vi "LS370_setup.vi"   [LabVIEW 2016]
uses:
  Instrument_Setup.vi
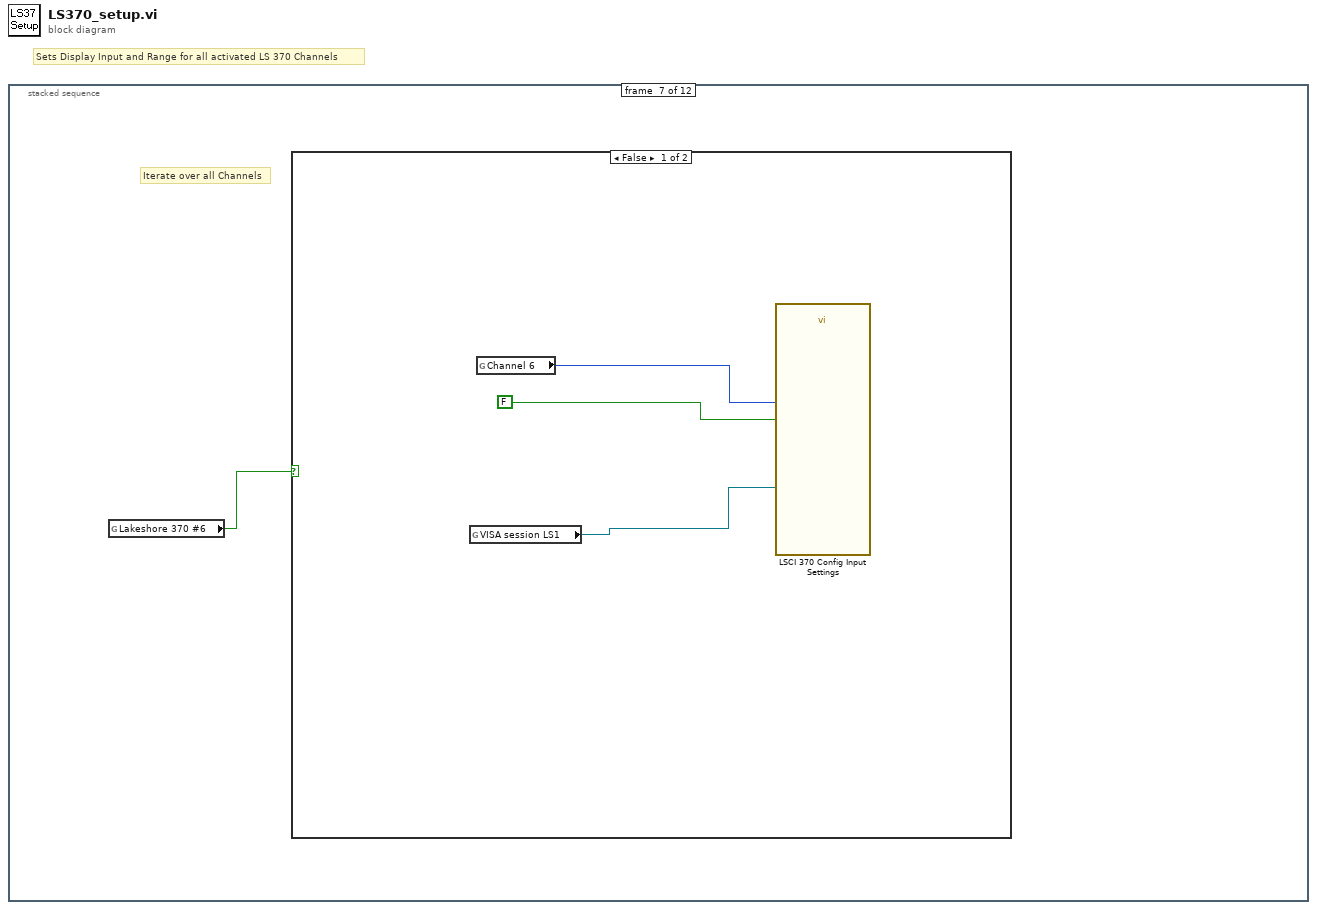
[diagram p0: block diagram]
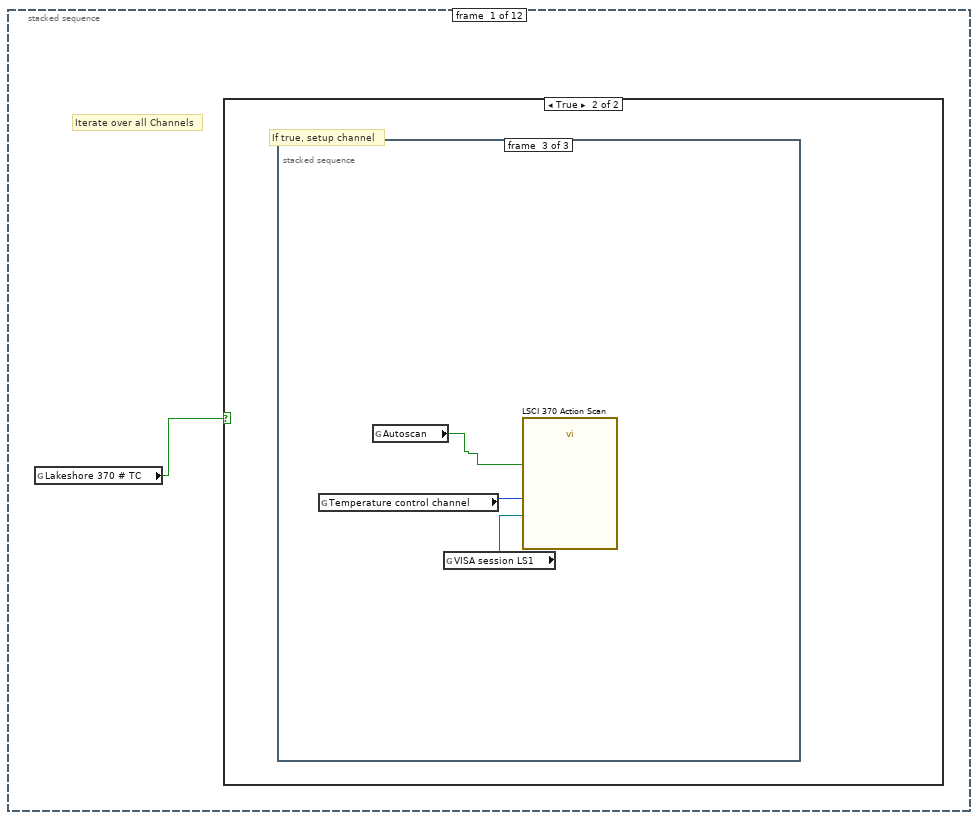
[diagram p2: hidden frame]
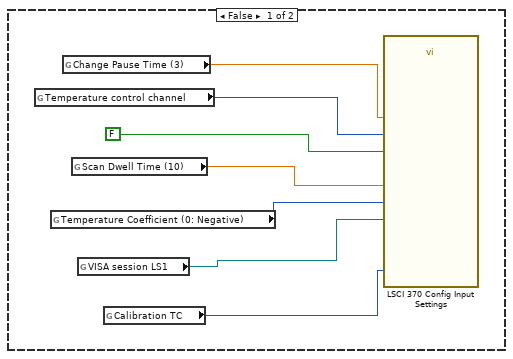
[diagram p3: hidden frame]
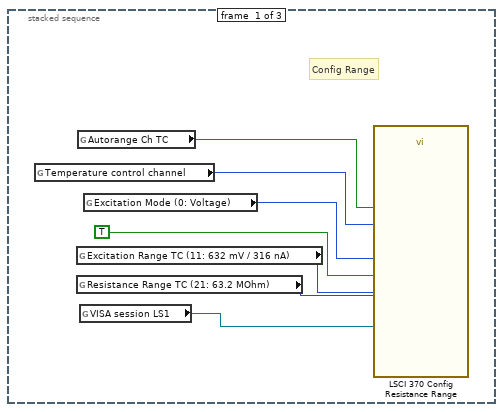
[diagram p4: hidden frame]
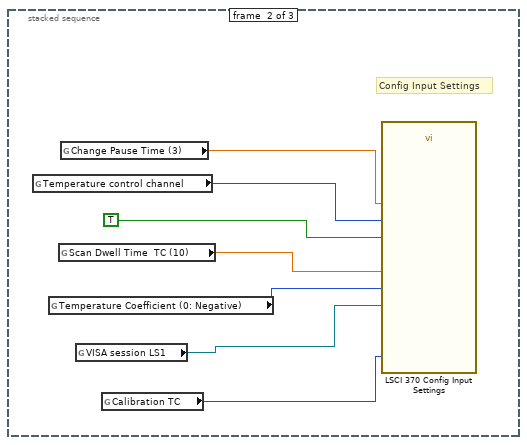
[diagram p5: hidden frame]
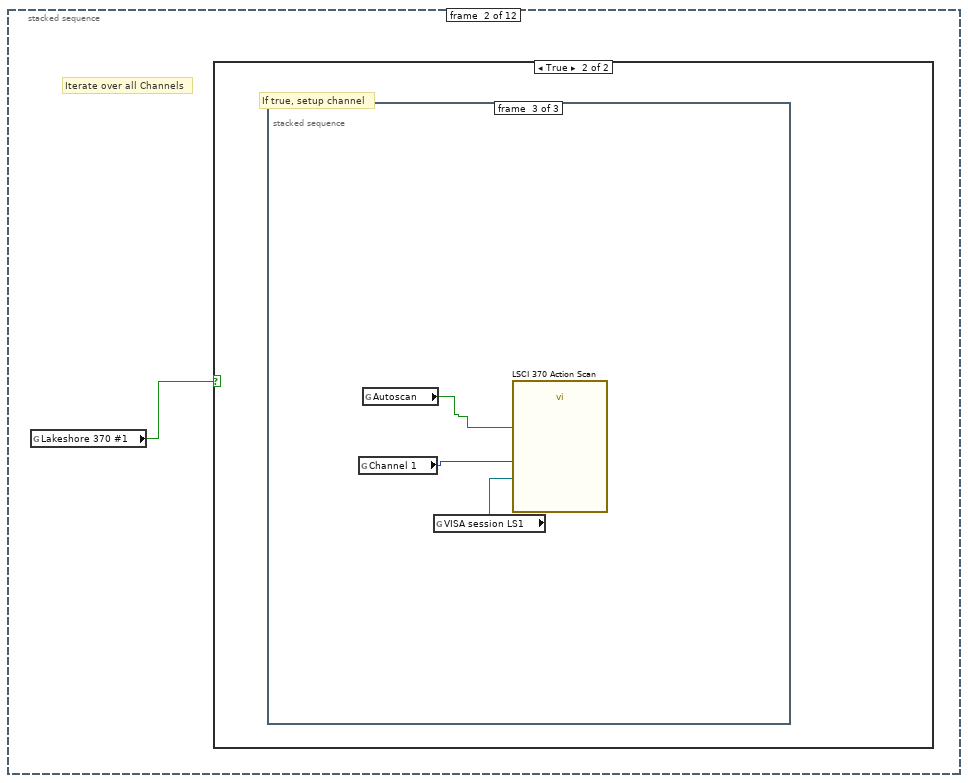
[diagram p6: hidden frame]
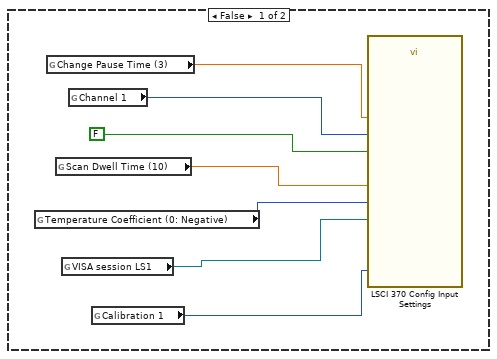
[diagram p7: hidden frame]
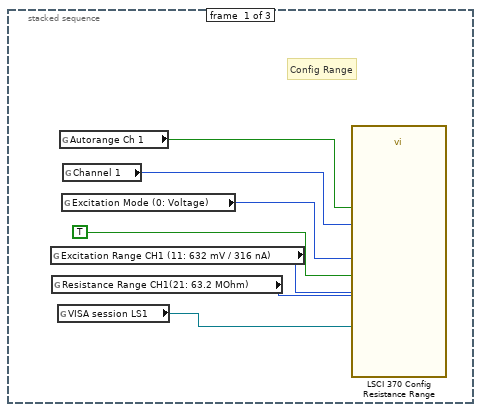
[diagram p8: hidden frame]
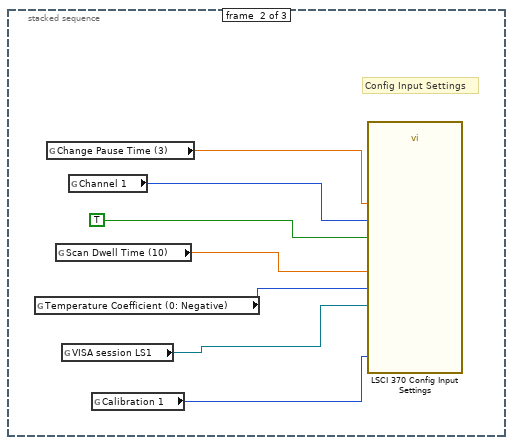
[diagram p9: hidden frame]
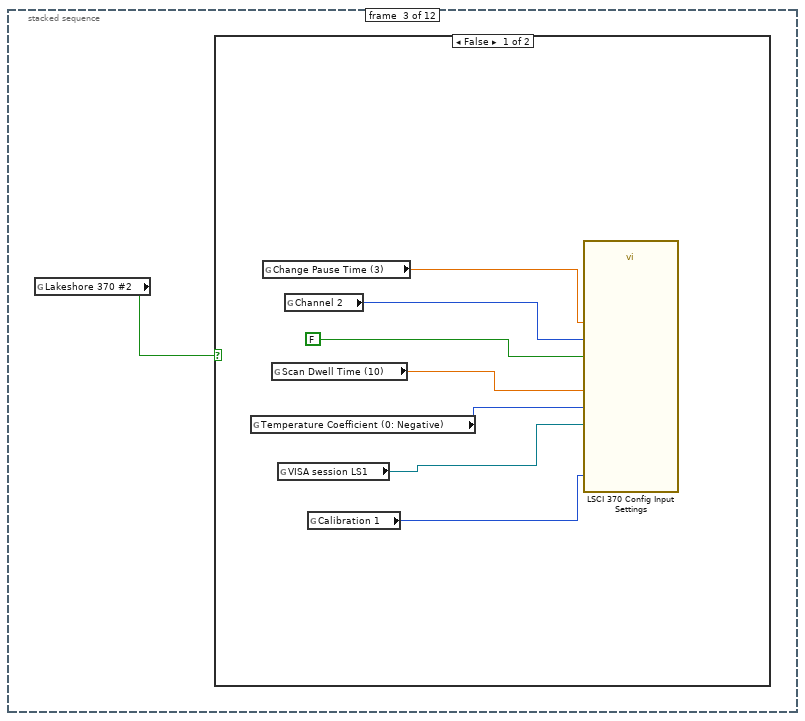
[diagram p10: hidden frame]
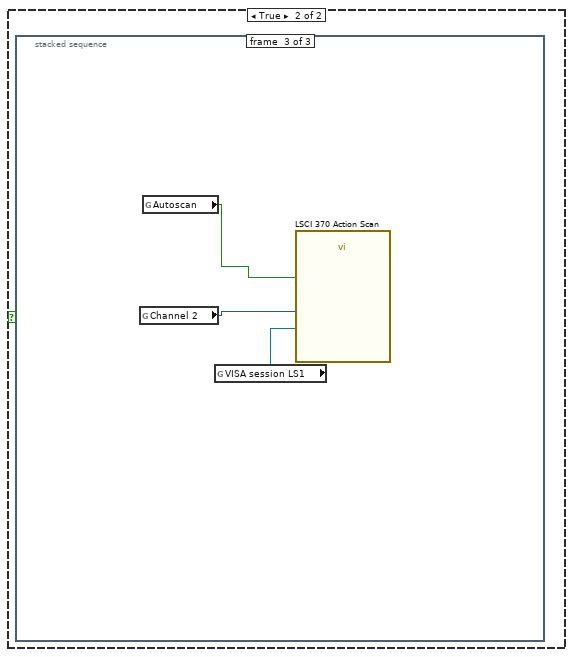
[diagram p11: hidden frame]
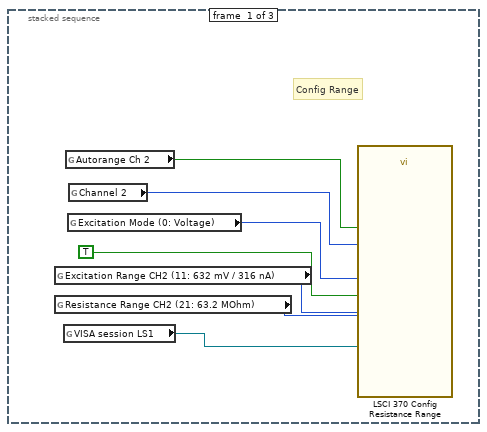
[diagram p12: hidden frame]
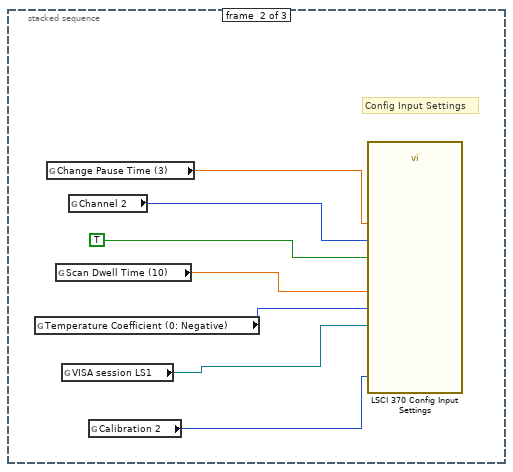
[diagram p13: hidden frame]
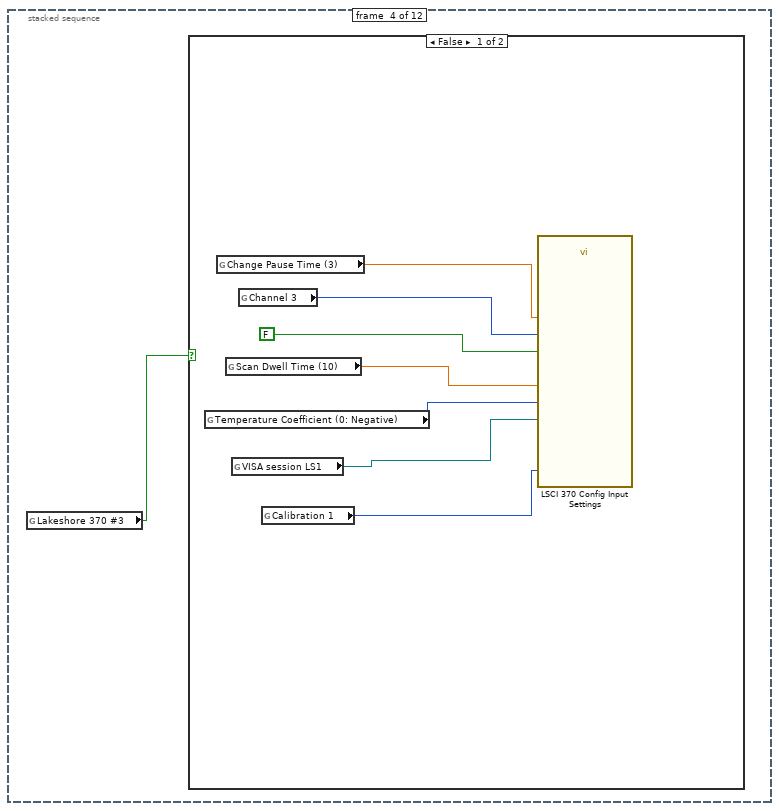
[diagram p14: hidden frame]
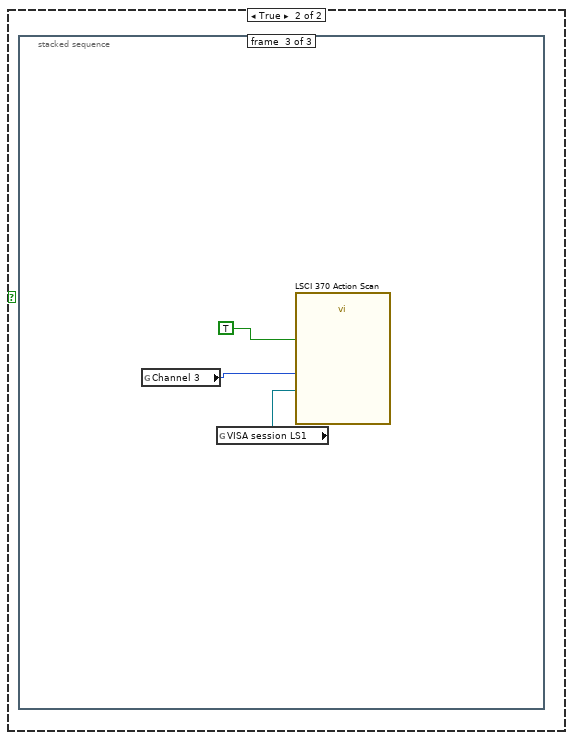
[diagram p15: hidden frame]
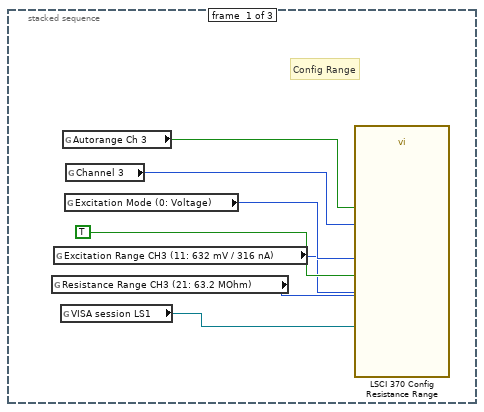
[diagram p16: hidden frame]
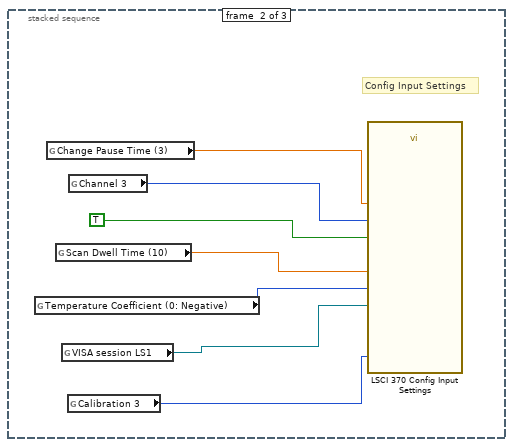
[diagram p17: hidden frame]
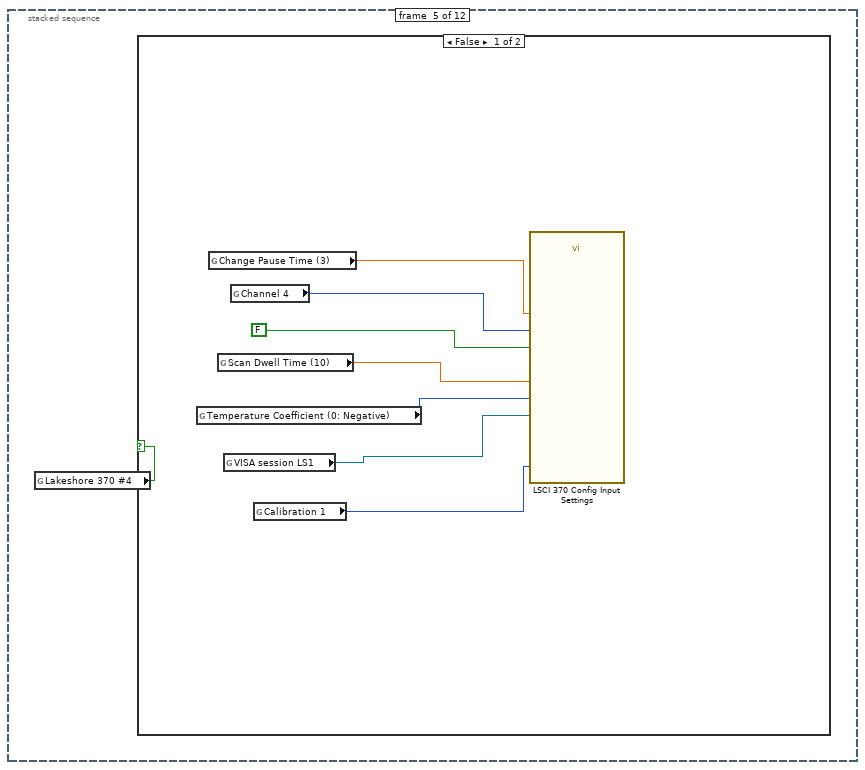
[diagram p18: hidden frame]
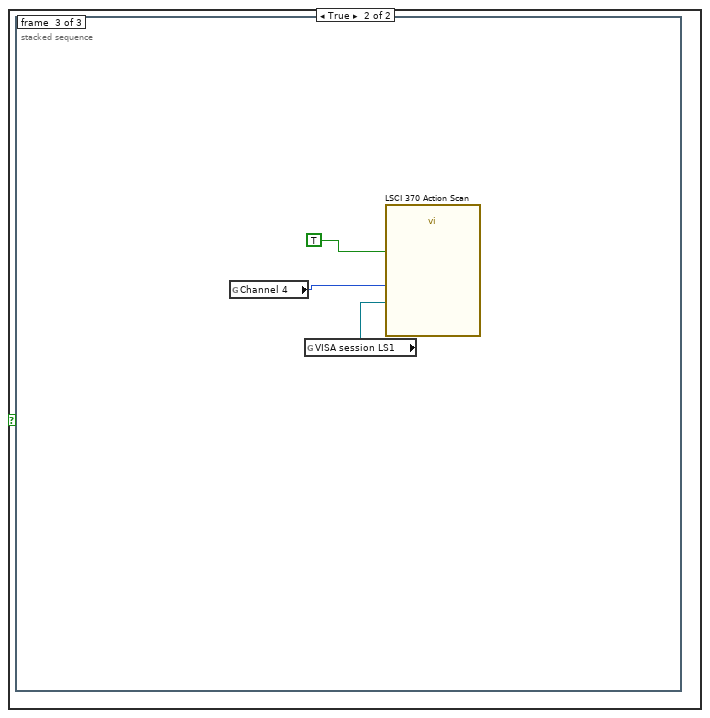
[diagram p19: hidden frame]
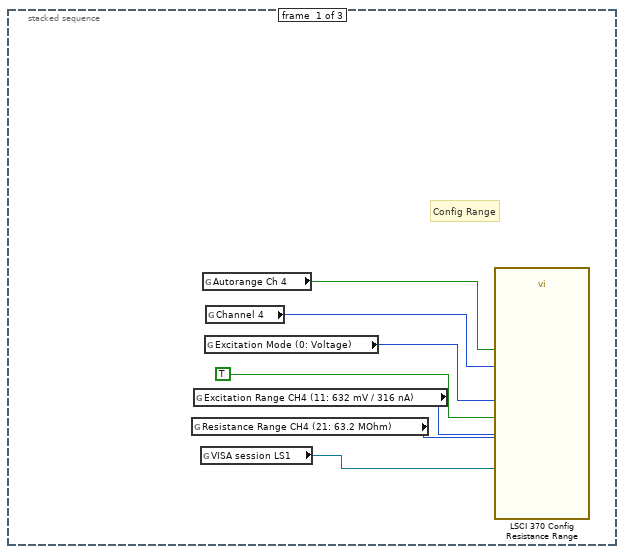
[diagram p20: hidden frame]
diagram:
  # "Sets Display Input and Range for all activated LS 370 Channels"
  n1 = stacked-sequence {
    frame #0 {
      # "Iterate over all Channels"
      n2 = global read "Instrument_Setup.vi" "Lakeshore 370 # TC"() -> (w1:bool)
      n3 = case shown="True" w1 {
        frame False {
          n4 = global read "Instrument_Setup.vi" "Temperature control channel"() -> (w2:i32)
          n5 = global read "Instrument_Setup.vi" "Temperature Coefficient (0: Negative)"() -> (w4:u16)
          n6 = global read "Instrument_Setup.vi" "Change Pause Time (3)"() -> (w8:dbl)
          n7 = global read "Instrument_Setup.vi" "Scan Dwell Time (10)"() -> (w6:dbl)
          n8 = global read "Instrument_Setup.vi" "VISA session LS1"() -> (w5:refnum<visa-resource-name>)
          n9 = global read "Instrument_Setup.vi" "Calibration TC"() -> (w3:i32)
          n10 = call "LSCI 370 Config Input Settings.vi"("VISA session"=w5, "Scan Dwell Time (10)"=w6, "Change Pause Time (3)"=w8, "Channel (1)"=w2, "Channel On/Off (T: Channel ON)"=FALSE, "Curve Number"=w3, "Temperature Coefficient (0: Negative)"=w4) -> ()  [unwired: 7 in, 2 out]
        }
        frame True {
          # "If true, setup channel"
          n11 = stacked-sequence {
            frame #0 {
              # "Config Range"
              n12 = global read "Instrument_Setup.vi" "Temperature control channel"() -> (w11:i32)
              n13 = global read "Instrument_Setup.vi" "Excitation Range TC (11: 632 mV / 316 nA)"() -> (w13:u16)
              n14 = global read "Instrument_Setup.vi" "Resistance Range TC (21: 63.2 MOhm)"() -> (w14:u16)
              n15 = global read "Instrument_Setup.vi" "Autorange Ch TC"() -> (w10:bool)
              n16 = global read "Instrument_Setup.vi" "VISA session LS1"() -> (w15:refnum<visa-resource-name>)
              n17 = global read "Instrument_Setup.vi" "Excitation Mode (0: Voltage)"() -> (w12:u16)
              n18 = call "LSCI 370 Config Resistance Range.vi"("VISA session"=w15, "Autorange (F: Autorange OFF)"=w10, "Excitation On/Off (T: Excitation ON)"=TRUE, "Channel (1)"=w11, "Excitation Mode (0: Voltage)"=w12, "Excitation Range (11: 632 mV / 316 nA)"=w13, "Resistance Range (21: 63.2 MOhm)"=w14) -> ()  [unwired: 7 in, 2 out]
            }
            frame #1 {
              # "Config Input Settings"
              n19 = global read "Instrument_Setup.vi" "Temperature control channel"() -> (w21:i32)
              n20 = global read "Instrument_Setup.vi" "Temperature Coefficient (0: Negative)"() -> (w17:u16)
              n21 = global read "Instrument_Setup.vi" "Scan Dwell Time  TC (10)"() -> (w19:dbl)
              n22 = global read "Instrument_Setup.vi" "Change Pause Time (3)"() -> (w22:dbl)
              n23 = global read "Instrument_Setup.vi" "VISA session LS1"() -> (w18:refnum<visa-resource-name>)
              n24 = global read "Instrument_Setup.vi" "Calibration TC"() -> (w16:i32)
              n25 = call "LSCI 370 Config Input Settings.vi"("VISA session"=w18, "Scan Dwell Time (10)"=w19, "Change Pause Time (3)"=w22, "Channel (1)"=w21, "Channel On/Off (T: Channel ON)"=TRUE, "Curve Number"=w16, "Temperature Coefficient (0: Negative)"=w17) -> ()  [unwired: 7 in, 2 out]
            }
            frame #2 {
              n26 = global read "Instrument_Setup.vi" "Temperature control channel"() -> (w24:i32)
              n27 = global read "Instrument_Setup.vi" "Autoscan"() -> (w23:bool)
              n28 = global read "Instrument_Setup.vi" "VISA session LS1"() -> (w25:refnum<visa-resource-name>)
              n29 = call "LSCI 370 Action Scan.vi"("VISA session"=w25, "Scan Channel (1)"=w24, "Autoscan (F: Autoscan Off)"=w23) -> ()  [unwired: 11 in, 2 out]
            }
          }
        }
      }
    }
    frame #1 {
      # "Iterate over all Channels"
      n30 = global read "Instrument_Setup.vi" "Lakeshore 370 #1"() -> (w26:bool)
      n31 = case shown="True" w26 {
        frame False {
          n32 = global read "Instrument_Setup.vi" "Temperature Coefficient (0: Negative)"() -> (w29:u16)
          n33 = global read "Instrument_Setup.vi" "Change Pause Time (3)"() -> (w33:dbl)
          n34 = global read "Instrument_Setup.vi" "Scan Dwell Time (10)"() -> (w31:dbl)
          n35 = global read "Instrument_Setup.vi" "VISA session LS1"() -> (w30:refnum<visa-resource-name>)
          n36 = global read "Instrument_Setup.vi" "Channel 1"() -> (w27:i32)
          n37 = global read "Instrument_Setup.vi" "Calibration 1"() -> (w28:i32)
          n38 = call "LSCI 370 Config Input Settings.vi"("VISA session"=w30, "Scan Dwell Time (10)"=w31, "Change Pause Time (3)"=w33, "Channel (1)"=w27, "Channel On/Off (T: Channel ON)"=FALSE, "Curve Number"=w28, "Temperature Coefficient (0: Negative)"=w29) -> ()  [unwired: 7 in, 2 out]
        }
        frame True {
          # "If true, setup channel"
          n39 = stacked-sequence {
            frame #0 {
              # "Config Range"
              n40 = global read "Instrument_Setup.vi" "Excitation Range CH1 (11: 632 mV / 316 nA)"() -> (w38:u16)
              n41 = global read "Instrument_Setup.vi" "Resistance Range CH1(21: 63.2 MOhm)"() -> (w39:u16)
              n42 = global read "Instrument_Setup.vi" "VISA session LS1"() -> (w40:refnum<visa-resource-name>)
              n43 = global read "Instrument_Setup.vi" "Autorange Ch 1"() -> (w35:bool)
              n44 = global read "Instrument_Setup.vi" "Excitation Mode (0: Voltage)"() -> (w37:u16)
              n45 = global read "Instrument_Setup.vi" "Channel 1"() -> (w36:i32)
              n46 = call "LSCI 370 Config Resistance Range.vi"("VISA session"=w40, "Autorange (F: Autorange OFF)"=w35, "Excitation On/Off (T: Excitation ON)"=TRUE, "Channel (1)"=w36, "Excitation Mode (0: Voltage)"=w37, "Excitation Range (11: 632 mV / 316 nA)"=w38, "Resistance Range (21: 63.2 MOhm)"=w39) -> ()  [unwired: 7 in, 2 out]
            }
            frame #1 {
              # "Config Input Settings"
              n47 = global read "Instrument_Setup.vi" "Temperature Coefficient (0: Negative)"() -> (w42:u16)
              n48 = global read "Instrument_Setup.vi" "Change Pause Time (3)"() -> (w47:dbl)
              n49 = global read "Instrument_Setup.vi" "Scan Dwell Time (10)"() -> (w44:dbl)
              n50 = global read "Instrument_Setup.vi" "VISA session LS1"() -> (w43:refnum<visa-resource-name>)
              n51 = global read "Instrument_Setup.vi" "Channel 1"() -> (w46:i32)
              n52 = global read "Instrument_Setup.vi" "Calibration 1"() -> (w41:i32)
              n53 = call "LSCI 370 Config Input Settings.vi"("VISA session"=w43, "Scan Dwell Time (10)"=w44, "Change Pause Time (3)"=w47, "Channel (1)"=w46, "Channel On/Off (T: Channel ON)"=TRUE, "Curve Number"=w41, "Temperature Coefficient (0: Negative)"=w42) -> ()  [unwired: 7 in, 2 out]
            }
            frame #2 {
              n54 = global read "Instrument_Setup.vi" "Channel 1"() -> (w49:i32)
              n55 = global read "Instrument_Setup.vi" "Autoscan"() -> (w48:bool)
              n56 = global read "Instrument_Setup.vi" "VISA session LS1"() -> (w50:refnum<visa-resource-name>)
              n57 = call "LSCI 370 Action Scan.vi"("VISA session"=w50, "Scan Channel (1)"=w49, "Autoscan (F: Autoscan Off)"=w48) -> ()  [unwired: 11 in, 2 out]
            }
          }
        }
      }
    }
    frame #2 {
      n58 = global read "Instrument_Setup.vi" "Lakeshore 370 #2"() -> (w51:bool)
      n59 = case shown="False" w51 {
        frame False {
          n60 = global read "Instrument_Setup.vi" "Temperature Coefficient (0: Negative)"() -> (w53:u16)
          n61 = global read "Instrument_Setup.vi" "Change Pause Time (3)"() -> (w58:dbl)
          n62 = global read "Instrument_Setup.vi" "Scan Dwell Time (10)"() -> (w55:dbl)
          n63 = global read "Instrument_Setup.vi" "VISA session LS1"() -> (w54:refnum<visa-resource-name>)
          n64 = global read "Instrument_Setup.vi" "Channel 2"() -> (w57:i32)
          n65 = global read "Instrument_Setup.vi" "Calibration 1"() -> (w52:i32)
          n66 = call "LSCI 370 Config Input Settings.vi"("VISA session"=w54, "Scan Dwell Time (10)"=w55, "Change Pause Time (3)"=w58, "Channel (1)"=w57, "Channel On/Off (T: Channel ON)"=FALSE, "Curve Number"=w52, "Temperature Coefficient (0: Negative)"=w53) -> ()  [unwired: 7 in, 2 out]
        }
        frame True {
          n67 = stacked-sequence {
            frame #0 {
              # "Config Range"
              n68 = global read "Instrument_Setup.vi" "Excitation Range CH2 (11: 632 mV / 316 nA)"() -> (w63:u16)
              n69 = global read "Instrument_Setup.vi" "Resistance Range CH2 (21: 63.2 MOhm)"() -> (w64:u16)
              n70 = global read "Instrument_Setup.vi" "VISA session LS1"() -> (w65:refnum<visa-resource-name>)
              n71 = global read "Instrument_Setup.vi" "Autorange Ch 2"() -> (w60:bool)
              n72 = global read "Instrument_Setup.vi" "Excitation Mode (0: Voltage)"() -> (w62:u16)
              n73 = global read "Instrument_Setup.vi" "Channel 2"() -> (w61:i32)
              n74 = call "LSCI 370 Config Resistance Range.vi"("VISA session"=w65, "Autorange (F: Autorange OFF)"=w60, "Excitation On/Off (T: Excitation ON)"=TRUE, "Channel (1)"=w61, "Excitation Mode (0: Voltage)"=w62, "Excitation Range (11: 632 mV / 316 nA)"=w63, "Resistance Range (21: 63.2 MOhm)"=w64) -> ()  [unwired: 7 in, 2 out]
            }
            frame #1 {
              # "Config Input Settings"
              n75 = global read "Instrument_Setup.vi" "Temperature Coefficient (0: Negative)"() -> (w67:u16)
              n76 = global read "Instrument_Setup.vi" "Change Pause Time (3)"() -> (w72:dbl)
              n77 = global read "Instrument_Setup.vi" "Scan Dwell Time (10)"() -> (w69:dbl)
              n78 = global read "Instrument_Setup.vi" "VISA session LS1"() -> (w68:refnum<visa-resource-name>)
              n79 = global read "Instrument_Setup.vi" "Channel 2"() -> (w71:i32)
              n80 = global read "Instrument_Setup.vi" "Calibration 2"() -> (w66:i32)
              n81 = call "LSCI 370 Config Input Settings.vi"("VISA session"=w68, "Scan Dwell Time (10)"=w69, "Change Pause Time (3)"=w72, "Channel (1)"=w71, "Channel On/Off (T: Channel ON)"=TRUE, "Curve Number"=w66, "Temperature Coefficient (0: Negative)"=w67) -> ()  [unwired: 7 in, 2 out]
            }
            frame #2 {
              n82 = global read "Instrument_Setup.vi" "Channel 2"() -> (w74:i32)
              n83 = global read "Instrument_Setup.vi" "Autoscan"() -> (w73:bool)
              n84 = global read "Instrument_Setup.vi" "VISA session LS1"() -> (w75:refnum<visa-resource-name>)
              n85 = call "LSCI 370 Action Scan.vi"("VISA session"=w75, "Scan Channel (1)"=w74, "Autoscan (F: Autoscan Off)"=w73) -> ()  [unwired: 11 in, 2 out]
            }
          }
        }
      }
    }
    frame #3 {
      n86 = global read "Instrument_Setup.vi" "Lakeshore 370 #3"() -> (w76:bool)
      n87 = case shown="False" w76 {
        frame False {
          n88 = global read "Instrument_Setup.vi" "Temperature Coefficient (0: Negative)"() -> (w78:u16)
          n89 = global read "Instrument_Setup.vi" "Change Pause Time (3)"() -> (w83:dbl)
          n90 = global read "Instrument_Setup.vi" "Scan Dwell Time (10)"() -> (w80:dbl)
          n91 = global read "Instrument_Setup.vi" "VISA session LS1"() -> (w79:refnum<visa-resource-name>)
          n92 = global read "Instrument_Setup.vi" "Channel 3"() -> (w82:i32)
          n93 = global read "Instrument_Setup.vi" "Calibration 1"() -> (w77:i32)
          n94 = call "LSCI 370 Config Input Settings.vi"("VISA session"=w79, "Scan Dwell Time (10)"=w80, "Change Pause Time (3)"=w83, "Channel (1)"=w82, "Channel On/Off (T: Channel ON)"=FALSE, "Curve Number"=w77, "Temperature Coefficient (0: Negative)"=w78) -> ()  [unwired: 7 in, 2 out]
        }
        frame True {
          n95 = stacked-sequence {
            frame #0 {
              # "Config Range"
              n96 = global read "Instrument_Setup.vi" "Resistance Range CH3 (21: 63.2 MOhm)"() -> (w89:u16)
              n97 = global read "Instrument_Setup.vi" "Excitation Range CH3 (11: 632 mV / 316 nA)"() -> (w84:u16)
              n98 = global read "Instrument_Setup.vi" "VISA session LS1"() -> (w90:refnum<visa-resource-name>)
              n99 = global read "Instrument_Setup.vi" "Autorange Ch 3"() -> (w86:bool)
              n100 = global read "Instrument_Setup.vi" "Excitation Mode (0: Voltage)"() -> (w88:u16)
              n101 = global read "Instrument_Setup.vi" "Channel 3"() -> (w87:i32)
              n102 = call "LSCI 370 Config Resistance Range.vi"("VISA session"=w90, "Autorange (F: Autorange OFF)"=w86, "Excitation On/Off (T: Excitation ON)"=TRUE, "Channel (1)"=w87, "Excitation Mode (0: Voltage)"=w88, "Excitation Range (11: 632 mV / 316 nA)"=w84, "Resistance Range (21: 63.2 MOhm)"=w89) -> ()  [unwired: 7 in, 2 out]
            }
            frame #1 {
              # "Config Input Settings"
              n103 = global read "Instrument_Setup.vi" "Temperature Coefficient (0: Negative)"() -> (w92:u16)
              n104 = global read "Instrument_Setup.vi" "Change Pause Time (3)"() -> (w97:dbl)
              n105 = global read "Instrument_Setup.vi" "Scan Dwell Time (10)"() -> (w94:dbl)
              n106 = global read "Instrument_Setup.vi" "VISA session LS1"() -> (w93:refnum<visa-resource-name>)
              n107 = global read "Instrument_Setup.vi" "Calibration 3"() -> (w91:i32)
              n108 = global read "Instrument_Setup.vi" "Channel 3"() -> (w96:i32)
              n109 = call "LSCI 370 Config Input Settings.vi"("VISA session"=w93, "Scan Dwell Time (10)"=w94, "Change Pause Time (3)"=w97, "Channel (1)"=w96, "Channel On/Off (T: Channel ON)"=TRUE, "Curve Number"=w91, "Temperature Coefficient (0: Negative)"=w92) -> ()  [unwired: 7 in, 2 out]
            }
            frame #2 {
              n110 = global read "Instrument_Setup.vi" "Channel 3"() -> (w98:i32)
              n111 = global read "Instrument_Setup.vi" "VISA session LS1"() -> (w100:refnum<visa-resource-name>)
              n112 = call "LSCI 370 Action Scan.vi"("VISA session"=w100, "Scan Channel (1)"=w98, "Autoscan (F: Autoscan Off)"=TRUE) -> ()  [unwired: 11 in, 2 out]
            }
          }
        }
      }
    }
    frame #4 {
      n113 = global read "Instrument_Setup.vi" "Lakeshore 370 #4"() -> (w101:bool)
      n114 = case shown="False" w101 {
        frame False {
          n115 = global read "Instrument_Setup.vi" "Temperature Coefficient (0: Negative)"() -> (w103:u16)
          n116 = global read "Instrument_Setup.vi" "Change Pause Time (3)"() -> (w108:dbl)
          n117 = global read "Instrument_Setup.vi" "Scan Dwell Time (10)"() -> (w105:dbl)
          n118 = global read "Instrument_Setup.vi" "VISA session LS1"() -> (w104:refnum<visa-resource-name>)
          n119 = global read "Instrument_Setup.vi" "Channel 4"() -> (w107:i32)
          n120 = global read "Instrument_Setup.vi" "Calibration 1"() -> (w102:i32)
          n121 = call "LSCI 370 Config Input Settings.vi"("VISA session"=w104, "Scan Dwell Time (10)"=w105, "Change Pause Time (3)"=w108, "Channel (1)"=w107, "Channel On/Off (T: Channel ON)"=FALSE, "Curve Number"=w102, "Temperature Coefficient (0: Negative)"=w103) -> ()  [unwired: 7 in, 2 out]
        }
        frame True {
          n122 = stacked-sequence {
            frame #0 {
              # "Config Range"
              n123 = global read "Instrument_Setup.vi" "Resistance Range CH4 (21: 63.2 MOhm)"() -> (w114:u16)
              n124 = global read "Instrument_Setup.vi" "Excitation Range CH4 (11: 632 mV / 316 nA)"() -> (w113:u16)
              n125 = global read "Instrument_Setup.vi" "VISA session LS1"() -> (w115:refnum<visa-resource-name>)
              n126 = global read "Instrument_Setup.vi" "Autorange Ch 4"() -> (w110:bool)
              n127 = global read "Instrument_Setup.vi" "Excitation Mode (0: Voltage)"() -> (w112:u16)
              n128 = global read "Instrument_Setup.vi" "Channel 4"() -> (w111:i32)
              n129 = call "LSCI 370 Config Resistance Range.vi"("VISA session"=w115, "Autorange (F: Autorange OFF)"=w110, "Excitation On/Off (T: Excitation ON)"=TRUE, "Channel (1)"=w111, "Excitation Mode (0: Voltage)"=w112, "Excitation Range (11: 632 mV / 316 nA)"=w113, "Resistance Range (21: 63.2 MOhm)"=w114) -> ()  [unwired: 7 in, 2 out]
            }
            frame #1 {
              # "Config Input Settings"
              n130 = global read "Instrument_Setup.vi" "Temperature Coefficient (0: Negative)"() -> (w117:u16)
              n131 = global read "Instrument_Setup.vi" "Change Pause Time (3)"() -> (w122:dbl)
              n132 = global read "Instrument_Setup.vi" "Scan Dwell Time (10)"() -> (w119:dbl)
              n133 = global read "Instrument_Setup.vi" "VISA session LS1"() -> (w118:refnum<visa-resource-name>)
              n134 = global read "Instrument_Setup.vi" "Channel 4"() -> (w121:i32)
              n135 = global read "Instrument_Setup.vi" "Calibration 4"() -> (w116:i32)
              n136 = call "LSCI 370 Config Input Settings.vi"("VISA session"=w118, "Scan Dwell Time (10)"=w119, "Change Pause Time (3)"=w122, "Channel (1)"=w121, "Channel On/Off (T: Channel ON)"=TRUE, "Curve Number"=w116, "Temperature Coefficient (0: Negative)"=w117) -> ()  [unwired: 7 in, 2 out]
            }
            frame #2 {
              n137 = global read "Instrument_Setup.vi" "Channel 4"() -> (w123:i32)
              n138 = global read "Instrument_Setup.vi" "VISA session LS1"() -> (w125:refnum<visa-resource-name>)
              n139 = call "LSCI 370 Action Scan.vi"("VISA session"=w125, "Scan Channel (1)"=w123, "Autoscan (F: Autoscan Off)"=TRUE) -> ()  [unwired: 11 in, 2 out]
            }
          }
        }
      }
    }
    frame #5 {
      n140 = global read "Instrument_Setup.vi" "Lakeshore 370 #5"() -> (w126:bool)
      n141 = case shown="False" w126 {
        frame False {
          n142 = global read "Instrument_Setup.vi" "Temperature Coefficient (0: Negative)"() -> (w128:u16)
          n143 = global read "Instrument_Setup.vi" "Change Pause Time (3)"() -> (w133:dbl)
          n144 = global read "Instrument_Setup.vi" "Scan Dwell Time (10)"() -> (w130:dbl)
          n145 = global read "Instrument_Setup.vi" "VISA session LS1"() -> (w129:refnum<visa-resource-name>)
          n146 = global read "Instrument_Setup.vi" "Channel 5"() -> (w132:i32)
          n147 = global read "Instrument_Setup.vi" "Calibration 1"() -> (w127:i32)
          n148 = call "LSCI 370 Config Input Settings.vi"("VISA session"=w129, "Scan Dwell Time (10)"=w130, "Change Pause Time (3)"=w133, "Channel (1)"=w132, "Channel On/Off (T: Channel ON)"=FALSE, "Curve Number"=w127, "Temperature Coefficient (0: Negative)"=w128) -> ()  [unwired: 7 in, 2 out]
        }
        frame True {
          n149 = stacked-sequence {
            frame #0 {
              # "Config Range"
              n150 = global read "Instrument_Setup.vi" "Excitation Range CH 5 (11: 632 mV / 316 nA)"() -> (w138:u16)
              n151 = global read "Instrument_Setup.vi" "Resistance Range CH5 (21: 63.2 MOhm)"() -> (w139:u16)
              n152 = global read "Instrument_Setup.vi" "VISA session LS1"() -> (w140:refnum<visa-resource-name>)
              n153 = global read "Instrument_Setup.vi" "Autorange Ch 5"() -> (w135:bool)
              n154 = global read "Instrument_Setup.vi" "Excitation Mode (0: Voltage)"() -> (w137:u16)
              n155 = global read "Instrument_Setup.vi" "Channel 5"() -> (w136:i32)
              n156 = call "LSCI 370 Config Resistance Range.vi"("VISA session"=w140, "Autorange (F: Autorange OFF)"=w135, "Excitation On/Off (T: Excitation ON)"=TRUE, "Channel (1)"=w136, "Excitation Mode (0: Voltage)"=w137, "Excitation Range (11: 632 mV / 316 nA)"=w138, "Resistance Range (21: 63.2 MOhm)"=w139) -> ()  [unwired: 7 in, 2 out]
            }
            frame #1 {
              # "Config Input Settings"
              n157 = global read "Instrument_Setup.vi" "Temperature Coefficient (0: Negative)"() -> (w142:u16)
              n158 = global read "Instrument_Setup.vi" "Change Pause Time (3)"() -> (w147:dbl)
              n159 = global read "Instrument_Setup.vi" "Scan Dwell Time (10)"() -> (w144:dbl)
              n160 = global read "Instrument_Setup.vi" "VISA session LS1"() -> (w143:refnum<visa-resource-name>)
              n161 = global read "Instrument_Setup.vi" "Channel 5"() -> (w146:i32)
              n162 = global read "Instrument_Setup.vi" "Calibration 5"() -> (w141:i32)
              n163 = call "LSCI 370 Config Input Settings.vi"("VISA session"=w143, "Scan Dwell Time (10)"=w144, "Change Pause Time (3)"=w147, "Channel (1)"=w146, "Channel On/Off (T: Channel ON)"=TRUE, "Curve Number"=w141, "Temperature Coefficient (0: Negative)"=w142) -> ()  [unwired: 7 in, 2 out]
            }
            frame #2 {
              n164 = global read "Instrument_Setup.vi" "Channel 5"() -> (w148:i32)
              n165 = global read "Instrument_Setup.vi" "VISA session LS1"() -> (w150:refnum<visa-resource-name>)
              n166 = call "LSCI 370 Action Scan.vi"("VISA session"=w150, "Scan Channel (1)"=w148, "Autoscan (F: Autoscan Off)"=TRUE) -> ()  [unwired: 11 in, 2 out]
            }
          }
        }
      }
    }
    frame #6 {
      # "Iterate over all Channels"
      n167 = global read "Instrument_Setup.vi" "Lakeshore 370 #6"() -> (w151:bool)
      n168 = case shown="False" w151 {
        frame False {
          n169 = global read "Instrument_Setup.vi" "VISA session LS1"() -> (w153:refnum<visa-resource-name>)
          n170 = global read "Instrument_Setup.vi" "Channel 6"() -> (w152:i32)
          n171 = call "LSCI 370 Config Input Settings.vi"("VISA session"=w153, "Channel (1)"=w152, "Channel On/Off (T: Channel ON)"=FALSE) -> ()  [unwired: 11 in, 2 out]
        }
        frame True {
          # "If true, setup channel"
          n172 = stacked-sequence {
            frame #0 {
              # "Config Range"
              n173 = global read "Instrument_Setup.vi" "Excitation Range CH6 (11: 632 mV / 316 nA)"() -> (w159:u16)
              n174 = global read "Instrument_Setup.vi" "Resistance Range CH6(21: 63.2 MOhm)"() -> (w160:u16)
              n175 = global read "Instrument_Setup.vi" "VISA session LS1"() -> (w161:refnum<visa-resource-name>)
              n176 = global read "Instrument_Setup.vi" "Autorange Ch 6"() -> (w156:bool)
              n177 = global read "Instrument_Setup.vi" "Excitation Mode (0: Voltage)"() -> (w158:u16)
              n178 = global read "Instrument_Setup.vi" "Channel 6"() -> (w157:i32)
              n179 = call "LSCI 370 Config Resistance Range.vi"("VISA session"=w161, "Autorange (F: Autorange OFF)"=w156, "Excitation On/Off (T: Excitation ON)"=TRUE, "Channel (1)"=w157, "Excitation Mode (0: Voltage)"=w158, "Excitation Range (11: 632 mV / 316 nA)"=w159, "Resistance Range (21: 63.2 MOhm)"=w160) -> ()  [unwired: 7 in, 2 out]
            }
            frame #1 {
              # "Config Input Settings"
              n180 = global read "Instrument_Setup.vi" "Temperature Coefficient (0: Negative)"() -> (w163:u16)
              n181 = global read "Instrument_Setup.vi" "Change Pause Time (3)"() -> (w168:dbl)
              n182 = global read "Instrument_Setup.vi" "Scan Dwell Time (10)"() -> (w165:dbl)
              n183 = global read "Instrument_Setup.vi" "VISA session LS1"() -> (w164:refnum<visa-resource-name>)
              n184 = global read "Instrument_Setup.vi" "Channel 6"() -> (w167:i32)
              n185 = global read "Instrument_Setup.vi" "Calibration 6"() -> (w162:i32)
              n186 = call "LSCI 370 Config Input Settings.vi"("VISA session"=w164, "Scan Dwell Time (10)"=w165, "Change Pause Time (3)"=w168, "Channel (1)"=w167, "Channel On/Off (T: Channel ON)"=TRUE, "Curve Number"=w162, "Temperature Coefficient (0: Negative)"=w163) -> ()  [unwired: 7 in, 2 out]
            }
            frame #2 {
              n187 = global read "Instrument_Setup.vi" "Channel 6"() -> (w170:i32)
              n188 = global read "Instrument_Setup.vi" "Autoscan"() -> (w169:bool)
              n189 = global read "Instrument_Setup.vi" "VISA session LS1"() -> (w171:refnum<visa-resource-name>)
              n190 = call "LSCI 370 Action Scan.vi"("VISA session"=w171, "Scan Channel (1)"=w170, "Autoscan (F: Autoscan Off)"=w169) -> ()  [unwired: 11 in, 2 out]
            }
          }
        }
      }
    }
    frame #7 {
      # "Iterate over all Channels"
      n191 = global read "Instrument_Setup.vi" "Lakeshore 370 #7"() -> (w172:bool)
      n192 = case shown="False" w172 {
        frame False {
          n193 = global read "Instrument_Setup.vi" "VISA session LS1"() -> (w174:refnum<visa-resource-name>)
          n194 = global read "Instrument_Setup.vi" "Channel 7"() -> (w173:i32)
          n195 = call "LSCI 370 Config Input Settings.vi"("VISA session"=w174, "Channel (1)"=w173, "Channel On/Off (T: Channel ON)"=FALSE) -> ()  [unwired: 11 in, 2 out]
        }
        frame True {
          # "If true, setup channel"
          n196 = stacked-sequence {
            frame #0 {
              # "Config Range"
              n197 = global read "Instrument_Setup.vi" "Excitation Range CH7 (11: 632 mV / 316 nA)"() -> (w180:u16)
              n198 = global read "Instrument_Setup.vi" "Resistance Range CH7 (21: 63.2 MOhm)"() -> (w181:u16)
              n199 = global read "Instrument_Setup.vi" "VISA session LS1"() -> (w182:refnum<visa-resource-name>)
              n200 = global read "Instrument_Setup.vi" "Autorange Ch 7"() -> (w177:bool)
              n201 = global read "Instrument_Setup.vi" "Excitation Mode (0: Voltage)"() -> (w179:u16)
              n202 = global read "Instrument_Setup.vi" "Channel 7"() -> (w178:i32)
              n203 = call "LSCI 370 Config Resistance Range.vi"("VISA session"=w182, "Autorange (F: Autorange OFF)"=w177, "Excitation On/Off (T: Excitation ON)"=TRUE, "Channel (1)"=w178, "Excitation Mode (0: Voltage)"=w179, "Excitation Range (11: 632 mV / 316 nA)"=w180, "Resistance Range (21: 63.2 MOhm)"=w181) -> ()  [unwired: 7 in, 2 out]
            }
            frame #1 {
              # "Config Input Settings"
              n204 = global read "Instrument_Setup.vi" "Temperature Coefficient (0: Negative)"() -> (w184:u16)
              n205 = global read "Instrument_Setup.vi" "Change Pause Time (3)"() -> (w189:dbl)
              n206 = global read "Instrument_Setup.vi" "Scan Dwell Time (10)"() -> (w186:dbl)
              n207 = global read "Instrument_Setup.vi" "VISA session LS1"() -> (w185:refnum<visa-resource-name>)
              n208 = global read "Instrument_Setup.vi" "Channel 7"() -> (w188:i32)
              n209 = global read "Instrument_Setup.vi" "Calibration 7"() -> (w183:i32)
              n210 = call "LSCI 370 Config Input Settings.vi"("VISA session"=w185, "Scan Dwell Time (10)"=w186, "Change Pause Time (3)"=w189, "Channel (1)"=w188, "Channel On/Off (T: Channel ON)"=TRUE, "Curve Number"=w183, "Temperature Coefficient (0: Negative)"=w184) -> ()  [unwired: 7 in, 2 out]
            }
            frame #2 {
              n211 = global read "Instrument_Setup.vi" "Channel 7"() -> (w191:i32)
              n212 = global read "Instrument_Setup.vi" "Autoscan"() -> (w190:bool)
              n213 = global read "Instrument_Setup.vi" "VISA session LS1"() -> (w192:refnum<visa-resource-name>)
              n214 = call "LSCI 370 Action Scan.vi"("VISA session"=w192, "Scan Channel (1)"=w191, "Autoscan (F: Autoscan Off)"=w190) -> ()  [unwired: 11 in, 2 out]
            }
          }
        }
      }
    }
    frame #8 {
      # "Iterate over all Channels"
      n215 = global read "Instrument_Setup.vi" "Lakeshore 370 #8"() -> (w193:bool)
      n216 = case shown="True" w193 {
        frame False {
          n217 = global read "Instrument_Setup.vi" "VISA session LS1"() -> (w195:refnum<visa-resource-name>)
          n218 = global read "Instrument_Setup.vi" "Channel 8"() -> (w194:i32)
          n219 = call "LSCI 370 Config Input Settings.vi"("VISA session"=w195, "Channel (1)"=w194, "Channel On/Off (T: Channel ON)"=FALSE) -> ()  [unwired: 11 in, 2 out]
        }
        frame True {
          # "If true, setup channel"
          n220 = stacked-sequence {
            frame #0 {
              # "Config Range"
              n221 = global read "Instrument_Setup.vi" "Excitation Range CH8 (11: 632 mV / 316 nA)"() -> (w201:u16)
              n222 = global read "Instrument_Setup.vi" "Resistance Range CH8(21: 63.2 MOhm)"() -> (w202:u16)
              n223 = global read "Instrument_Setup.vi" "VISA session LS1"() -> (w203:refnum<visa-resource-name>)
              n224 = global read "Instrument_Setup.vi" "Autorange Ch 8"() -> (w198:bool)
              n225 = global read "Instrument_Setup.vi" "Excitation Mode (0: Voltage)"() -> (w200:u16)
              n226 = global read "Instrument_Setup.vi" "Channel 8"() -> (w199:i32)
              n227 = call "LSCI 370 Config Resistance Range.vi"("VISA session"=w203, "Autorange (F: Autorange OFF)"=w198, "Excitation On/Off (T: Excitation ON)"=TRUE, "Channel (1)"=w199, "Excitation Mode (0: Voltage)"=w200, "Excitation Range (11: 632 mV / 316 nA)"=w201, "Resistance Range (21: 63.2 MOhm)"=w202) -> ()  [unwired: 7 in, 2 out]
            }
            frame #1 {
              # "Config Input Settings"
              n228 = global read "Instrument_Setup.vi" "Temperature Coefficient (0: Negative)"() -> (w205:u16)
              n229 = global read "Instrument_Setup.vi" "Change Pause Time (3)"() -> (w210:dbl)
              n230 = global read "Instrument_Setup.vi" "Scan Dwell Time (10)"() -> (w207:dbl)
              n231 = global read "Instrument_Setup.vi" "VISA session LS1"() -> (w206:refnum<visa-resource-name>)
              n232 = global read "Instrument_Setup.vi" "Channel 8"() -> (w209:i32)
              n233 = global read "Instrument_Setup.vi" "Calibration 8"() -> (w204:i32)
              n234 = call "LSCI 370 Config Input Settings.vi"("VISA session"=w206, "Scan Dwell Time (10)"=w207, "Change Pause Time (3)"=w210, "Channel (1)"=w209, "Channel On/Off (T: Channel ON)"=TRUE, "Curve Number"=w204, "Temperature Coefficient (0: Negative)"=w205) -> ()  [unwired: 7 in, 2 out]
            }
            frame #2 {
              n235 = global read "Instrument_Setup.vi" "Channel 8"() -> (w212:i32)
              n236 = global read "Instrument_Setup.vi" "Autoscan"() -> (w211:bool)
              n237 = global read "Instrument_Setup.vi" "VISA session LS1"() -> (w213:refnum<visa-resource-name>)
              n238 = call "LSCI 370 Action Scan.vi"("VISA session"=w213, "Scan Channel (1)"=w212, "Autoscan (F: Autoscan Off)"=w211) -> ()  [unwired: 11 in, 2 out]
            }
          }
        }
      }
    }
    frame #9 {
      # "Iterate over all Channels"
      n239 = global read "Instrument_Setup.vi" "Lakeshore 370 #9"() -> (w214:bool)
      n240 = case shown="True" w214 {
        frame False {
          n241 = global read "Instrument_Setup.vi" "VISA session LS1"() -> (w216:refnum<visa-resource-name>)
          n242 = global read "Instrument_Setup.vi" "Channel 9"() -> (w215:i32)
          n243 = call "LSCI 370 Config Input Settings.vi"("VISA session"=w216, "Channel (1)"=w215, "Channel On/Off (T: Channel ON)"=FALSE) -> ()  [unwired: 11 in, 2 out]
        }
        frame True {
          # "If true, setup channel"
          n244 = stacked-sequence {
            frame #0 {
              # "Config Range"
              n245 = global read "Instrument_Setup.vi" "Excitation Range CH9(11: 632 mV / 316 nA)"() -> (w222:u16)
              n246 = global read "Instrument_Setup.vi" "Resistance Range CH9(21: 63.2 MOhm)"() -> (w223:u16)
              n247 = global read "Instrument_Setup.vi" "VISA session LS1"() -> (w224:refnum<visa-resource-name>)
              n248 = global read "Instrument_Setup.vi" "Autorange Ch 9"() -> (w219:bool)
              n249 = global read "Instrument_Setup.vi" "Excitation Mode (0: Voltage)"() -> (w221:u16)
              n250 = global read "Instrument_Setup.vi" "Channel 9"() -> (w220:i32)
              n251 = call "LSCI 370 Config Resistance Range.vi"("VISA session"=w224, "Autorange (F: Autorange OFF)"=w219, "Excitation On/Off (T: Excitation ON)"=TRUE, "Channel (1)"=w220, "Excitation Mode (0: Voltage)"=w221, "Excitation Range (11: 632 mV / 316 nA)"=w222, "Resistance Range (21: 63.2 MOhm)"=w223) -> ()  [unwired: 7 in, 2 out]
            }
            frame #1 {
              # "Config Input Settings"
              n252 = global read "Instrument_Setup.vi" "Temperature Coefficient (0: Negative)"() -> (w226:u16)
              n253 = global read "Instrument_Setup.vi" "Change Pause Time (3)"() -> (w231:dbl)
              n254 = global read "Instrument_Setup.vi" "Scan Dwell Time (10)"() -> (w228:dbl)
              n255 = global read "Instrument_Setup.vi" "VISA session LS1"() -> (w227:refnum<visa-resource-name>)
              n256 = global read "Instrument_Setup.vi" "Channel 9"() -> (w230:i32)
              n257 = global read "Instrument_Setup.vi" "Calibration 9"() -> (w225:i32)
              n258 = call "LSCI 370 Config Input Settings.vi"("VISA session"=w227, "Scan Dwell Time (10)"=w228, "Change Pause Time (3)"=w231, "Channel (1)"=w230, "Channel On/Off (T: Channel ON)"=TRUE, "Curve Number"=w225, "Temperature Coefficient (0: Negative)"=w226) -> ()  [unwired: 7 in, 2 out]
            }
            frame #2 {
              n259 = global read "Instrument_Setup.vi" "Channel 9"() -> (w233:i32)
              n260 = global read "Instrument_Setup.vi" "Autoscan"() -> (w232:bool)
              n261 = global read "Instrument_Setup.vi" "VISA session LS1"() -> (w234:refnum<visa-resource-name>)
              n262 = call "LSCI 370 Action Scan.vi"("VISA session"=w234, "Scan Channel (1)"=w233, "Autoscan (F: Autoscan Off)"=w232) -> ()  [unwired: 11 in, 2 out]
            }
          }
        }
      }
    }
    frame #10 {
      # "Set Zone Tuning"
      n263 = call "set_zone_properties.vi"() -> ()  [unwired: 1 in]
    }
    frame #11 {
      w241 = u16 6 items=["31.6 uA", "100 uA", "316 uA", "1.00 mA", "3.16 mA", "10.0 mA", "31.6 mA", "100 mA"] ("Maximum Heater Range (0: 31.6 uA)")
      w239 = u16 1 items=["Current", "Power"] ("Heater Output Display (0: Current)")
      w238 = u16 0 items=["Unfiltered", "Filtered"] ("Filtered Readings (0: Unfiltered)")
      w237 = u16 1 items=["Closed Loop PID", "Zone Tuning", "Open Loop", "Off"] ("Control Mode (0: Closed Loop PID)")
      # "Set Zone Tuning"
      n264 = global read "Instrument_Setup.vi" "Temperature control channel"() -> (w236:i32)
      n265 = global read "Instrument_Setup.vi" "VISA session LS1"() -> (w242:refnum<visa-resource-name>)
      n266 = Wait (ms)(milliseconds to wait=1) -> ()  [unwired: 1 out]
      n267 = call "LSCI 370 Config Control Mode.vi"("VISA session"=w242, "Control Mode (0: Closed Loop PID)"=w237, "Channel (1)"=w236, "Filtered Readings (0: Unfiltered)"=w238, "Heater Output Display (0: Current)"=w239, "Heater Resistance (100.00)"=500.0, "Maximum Heater Range (0: 31.6 uA)"=w241) -> ()  [unwired: 7 in, 2 out]
    }
  }
